vi "Set DC Pins.vi"(8 "error in (no error)":errorcluster, 11 "Harmonics in":refnum<class "Harmonics.lvclass">) -> (0 "error out":errorcluster, 3 "Harmonics out":refnum<class "Harmonics.lvclass">)   [LabVIEW 2018, in "Harmonics.lvlib" / "Harmonics.lvclass"]
uses:
  Harmonics.lvclass
  C:/Sequence Automation/Plugins/Measurement Interface.lvlibp/Measurement Interface.lvclass
  Harmonics.lvclass/Harmonics.ctl
  Protected Methods/Write DC Pins.vi
  Plugins/Measurement Interface.lvlibp/Private Methods/Measurement Parameters/Read Measurement Parameters.vi
  Plugins/String Database.lvlibp/String Database.lvclass
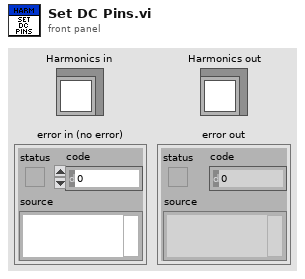
[diagram p1: front panel]
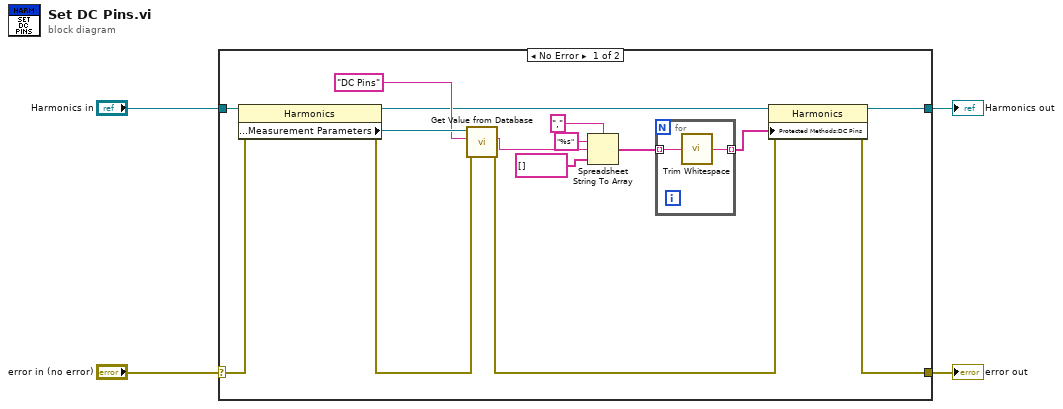
[diagram p0: block diagram]
diagram:
  n1 = case shown="No Error" "error in (no error)" {
    selector: "error in (no error)" -> [w19 w23]
    tunnel: [w8 w23] -> w3
    tunnel: [w6 w22] -> w1
    tunnel: "Harmonics in" -> [w18 w22]
    frame No Error {
      n2 = property class="Harmonics"(reference=w18, error in=w19) -> (reference out=w7:refnum<class "Harmonics.lvclass">, error out=w16:errorcluster, "Protected Methods:Measurement Parameters"=w17:refnum<class "String Database.lvclass">)
      n3 = call "Get Value from Database.vi"("error in (no error)"=w16, "Entry Name"="DC Pins", "Message in"=w17) -> ("error out"=w15:errorcluster, "Entry Value"=w11:string)  [unwired: 5 in, 2 out]
      n4 = Spreadsheet String To Array(delimiter (Tab)=",", format string="%s", spreadsheet string=w11, array type (2D Dbl)=string[] []) -> (array=w9:string[])
      n5 = for {
        tunnel: w9 -> [w21] mode=indexing
        tunnel: [w20] -> w5 mode=indexing
        n6 = call <vilib>:"Trim Whitespace.vi"("string"=w21) -> ("trimmed string"=w20:string)  [unwired: 1 in]
      }
      n7 = property class="Harmonics"(reference=w7, error in=w15, "Protected Methods:DC Pins"=w5) -> (reference out=w6:refnum<class "Harmonics.lvclass">, error out=w8:errorcluster)
    }
    frame Error {
    }
  }
  "error out" <- w3
  "Harmonics out" <- w1
